vi "Notifier Performance Test.vi"() -> ()   [LabVIEW 2021]
panel:
  out "x-y":dbl format="%#_6p"
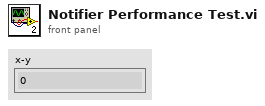
[diagram p1: front panel]
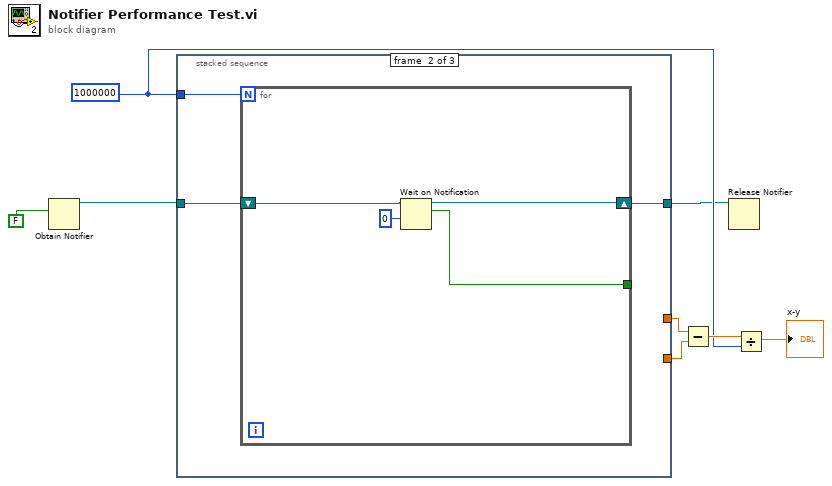
[diagram p0: block diagram]
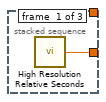
[diagram p2: hidden frame]
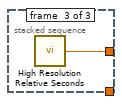
[diagram p3: hidden frame]
diagram:
  w4 = 1000000
  n1 = Obtain Notifier(notification data type=FALSE) -> (notifier out=w3:refnum<notifier>)  [unwired: 3 in, 2 out]
  n2 = stacked-sequence {
    tunnel: w3 -> [_ w12 _]
    tunnel: [_ w11 _] -> w1
    tunnel: [w9 _ _] -> w8
    tunnel: [_ _ w17] -> w7
    tunnel: w4 -> [_ w10 _]
    frame #0 {
      n3 = call <vilib>:"High Resolution Relative Seconds.vi"() -> ("relative seconds"=w9:dbl)
    }
    frame #1 {
      n4 = for {
        N: w10 -> [_]
        shift-right: [w15] -> w11
        shift-left: w12 -> [w16]
        tunnel: [w14] -> _
        n5 = Wait on Notification(notifier=w16, timeout in ms (-1)=0) -> (notifier out=w15:refnum<notifier>, notification=w14:bool)  [unwired: 2 in, 2 out]
      }
    }
    frame #2 {
      n6 = call <vilib>:"High Resolution Relative Seconds.vi"() -> ("relative seconds"=w17:dbl)
    }
  }
  n7 = Subtract(x=w7, y=w8) -> (x-y=w6:dbl)
  n8 = Release Notifier(notifier=w1) -> ()  [unwired: 2 in, 3 out]
  n9 = Divide(x=w6, y=w4) -> (x/y=→"x-y":dbl)
